vi "EndTestSuite_CallsListenerEndTestSuite.vi"() -> ()   [LabVIEW 2019, in "TestResultTest.lvlib"]
uses:
  TestResultTest.lvlib
  TestResult/TestResult.lvclass
  TestSuite/TestSuite.lvclass
  Support/FakeTestListener/FakeTestListener.lvclass
  C:/Users/de200256/Code/LVUnit/TestListener/TestListener.lvclass
  Assertion/Assertion.lvlib
panel:
  out "error out":errorcluster
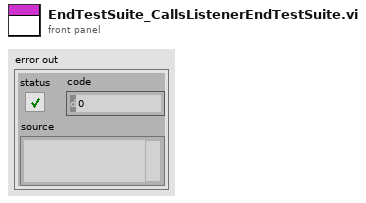
[diagram p1: front panel]
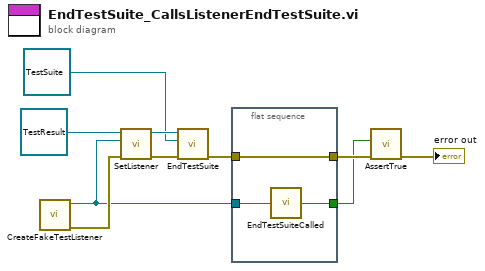
[diagram p0: block diagram]
diagram:
  n1 = call "CreateFakeTestListener.vi"() -> ("error out"=w9:errorcluster, "FakeTestListener"=w8:refnum<class "FakeTestListener.lvclass">)  [unwired: 10 in]
  n2 = call "SetListener.vi"("error in (no error)"=w9, "Listener"=w8, "TestResult in"=refnum<class "TestResult.lvclass"> refnum ("TestResult.lvclass")) -> ("error out"=w7:errorcluster, "TestResult in"=w5:refnum<class "TestResult.lvclass">)  [unwired: 7 in]
  n3 = call-dynamic "EndTestSuite.vi"("error in (no error)"=w7, "TestSuite"=refnum<class "TestSuite.lvclass"> refnum, "TestResult in"=w5) -> ("error out"=w6:errorcluster)  [unwired: 7 in, 1 out]
  n4 = flat-sequence {
    tunnel: w8 -> [w13]
    tunnel: w6 -> [w12]
    tunnel: [w12] -> w3
    tunnel: [w11] -> w2
    frame #0 {
      n5 = call "EndTestSuiteCalled.vi"("FakeTestListener In"=w13) -> ("EndTestSuite Called"=w11:bool)
    }
  }
  n6 = call "AssertTrue.vi"("error in (no error)"=w3, "Condition"=w2) -> ("error out"=→"error out":errorcluster)  [unwired: 9 in]
